vi "RT AND FPGA SETTINGS.vi"() -> ()   [LabVIEW 2018]
uses:
  Type Def Ctrls/RT ctrls/thermocouple type.ctl
panel:
  out "RT Main start time":string
  in  "ThermocoupleType":T1=6 items=["B", "E", "J", "K", "R", "S", "T", "N"]
  in  "FPGA I/O IRQ Number(s)":i32
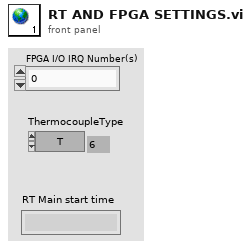
[diagram p1: front panel]
types:
  T1 = typedef "thermocouple type.ctl" = u16
diagram:
